vi "Destroy.vi"(8 "error in (no error)":errorcluster, 11 "WavBuf in":refnum<class "WavBuf.lvclass">) -> (0 "error out":errorcluster, 3 "WavBuf":refnum<class "WavBuf.lvclass">)   [LabVIEW 2025, in "WavBuf.lvclass"]
uses:
  WavBuf.lvclass
  WavBuf.lvclass/WavBuf.ctl
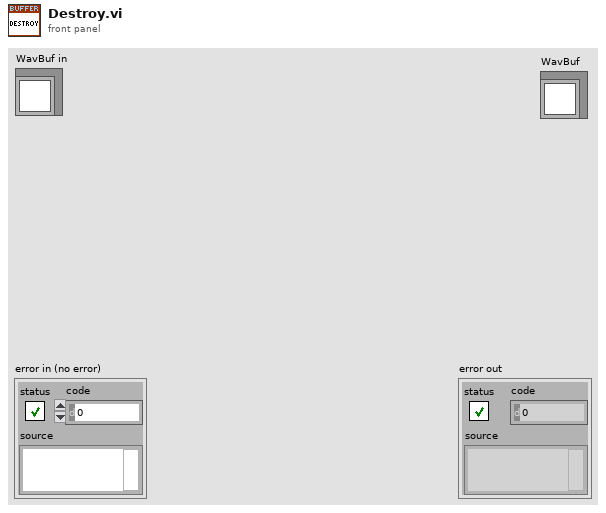
[diagram p1: front panel]
types:
  T1 = typedef "Ref_DVR_Buffer.ctl" = refnum<data-value>
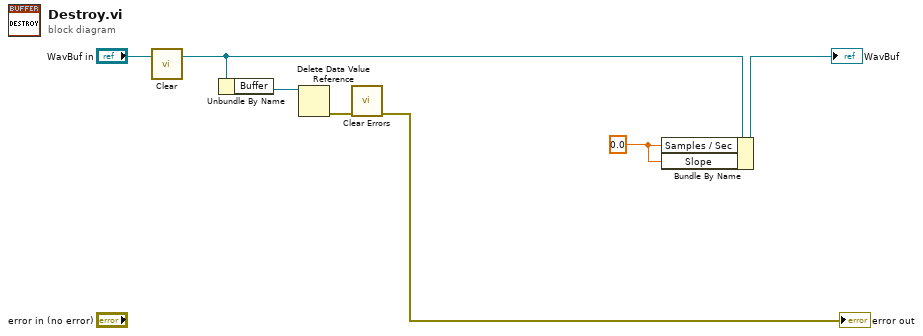
[diagram p0: block diagram]
diagram:
  w2 = 0.0 ("Samples / Sec")
  n1 = call-dynamic "Clear.vi"("WavBuf"="WavBuf in") -> ("WavBuf Out"=w1:refnum<class "WavBuf.lvclass">)  [unwired: 2 in]
  n2 = Unbundle By Name(w1) -> ("Buffer"=w5:T1)
  n3 = Delete Data Value Reference(data value reference=w5) -> (error out=w4:errorcluster)  [unwired: 1 in, 1 out]
  n4 = call <vilib>:"Clear Errors.vi"("error in (no error)"=w4) -> ("error out"=→"error out":errorcluster)  [unwired: 5 in, 1 out]
  n5 = Bundle By Name(cluster=w1, "Samples / Sec"=w2, "Slope"=w2) -> (→"WavBuf":refnum<class "WavBuf.lvclass">)
